vi "CmdControl _ch_1-12.vi"() -> (1 "Dataout":u8[](array[numeric]))   [LabVIEW 2017]
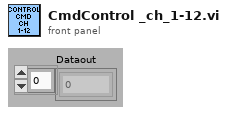
[diagram p1: front panel]
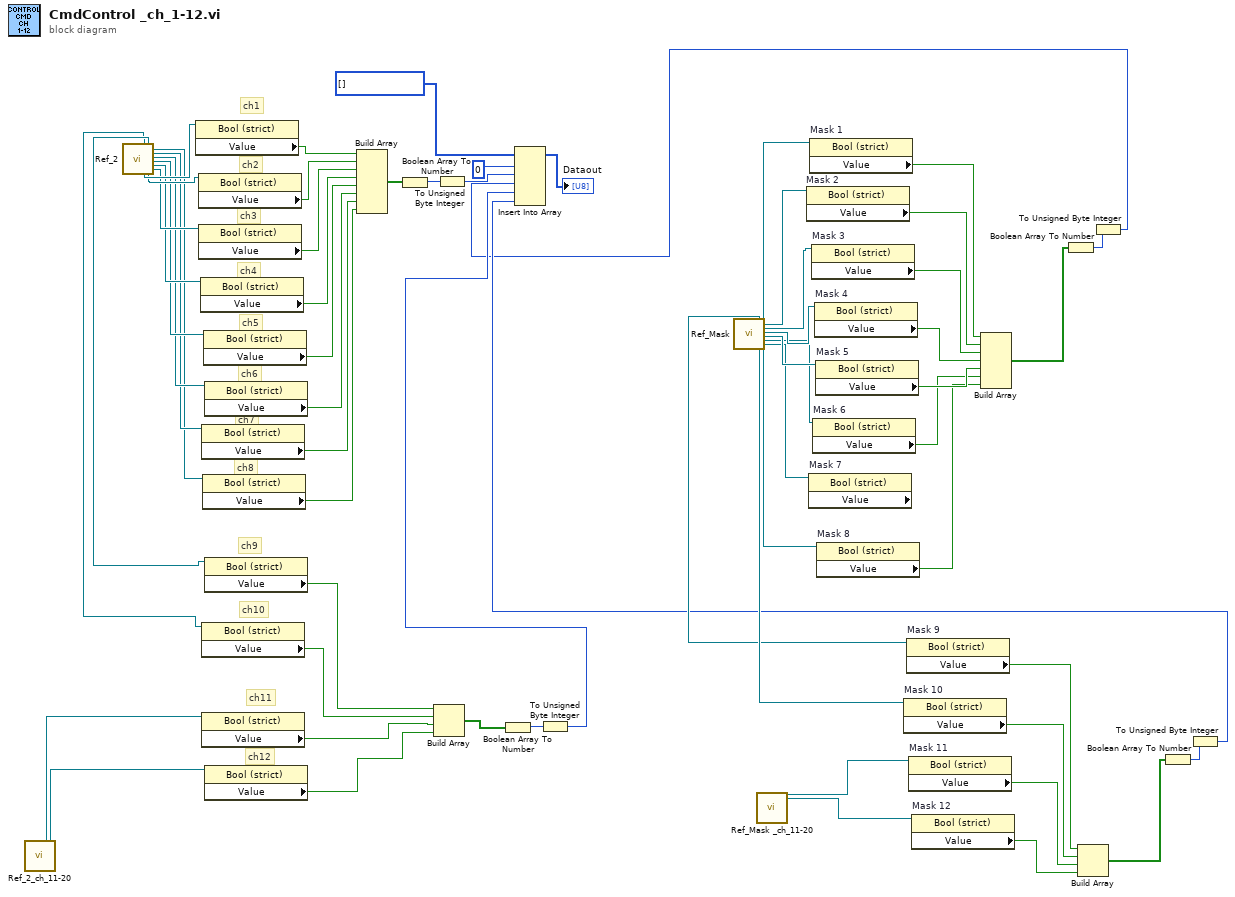
[diagram p0: block diagram]
diagram:
  # "ch12"
  # "ch11"
  # "ch10"
  # "ch9"
  # "ch8"
  # "ch7"
  # "ch6"
  # "ch5"
  # "ch4"
  # "ch3"
  # "ch2"
  # "ch1"
  n1 = call "Ref_2_ch_11-20.vi"() -> ("Control  Ch 11 out"=w37:refnum<vi>, "Control  Ch 12 out"=w38:refnum<vi>)  [unwired: 17 in, 9 out]
  n2 = call "Ref_2.vi"() -> ("Control  Ch 10 out"=w39:refnum<vi>, "Control  Ch 1 out"=w60:refnum<vi>, "Control  Ch 9 out"=w40:refnum<vi>, "Control  Ch 2 out"=w59:refnum<vi>, "Control  Ch 8 out"=w53:refnum<vi>, "Control  Ch 7 out"=w54:refnum<vi>, "Control  Ch 6 out"=w55:refnum<vi>, "Control  Ch 5 out"=w56:refnum<vi>, "Control  Ch 4 out"=w57:refnum<vi>, "Control  Ch 3 out"=w58:refnum<vi>)  [unwired: 17 in, 1 out]
  n3 = property class="Bool (strict)"(reference=w60) -> ("Value"=w52:bool)  [unwired: 1 in, 2 out]
  n4 = property class="Bool (strict)"(reference=w59) -> ("Value"=w51:bool)  [unwired: 1 in, 2 out]
  n5 = property class="Bool (strict)"(reference=w58) -> ("Value"=w50:bool)  [unwired: 1 in, 2 out]
  n6 = property class="Bool (strict)"(reference=w57) -> ("Value"=w49:bool)  [unwired: 1 in, 2 out]
  n7 = property class="Bool (strict)"(reference=w54) -> ("Value"=w46:bool)  [unwired: 1 in, 2 out]
  n8 = property class="Bool (strict)"(reference=w39) -> ("Value"=w35:bool)  [unwired: 1 in, 2 out]
  n9 = property class="Bool (strict)"(reference=w37) -> ("Value"=w34:bool)  [unwired: 1 in, 2 out]
  n10 = property class="Bool (strict)"(reference=w53) -> ("Value"=w45:bool)  [unwired: 1 in, 2 out]
  n11 = property class="Bool (strict)"(reference=w56) -> ("Value"=w48:bool)  [unwired: 1 in, 2 out]
  n12 = property class="Bool (strict)"(reference=w55) -> ("Value"=w47:bool)  [unwired: 1 in, 2 out]
  n13 = property class="Bool (strict)"(reference=w40) -> ("Value"=w36:bool)  [unwired: 1 in, 2 out]
  n14 = property class="Bool (strict)"(reference=w38) -> ("Value"=w33:bool)  [unwired: 1 in, 2 out]
  n15 = Build Array(w52, w51, w50, w49, w48, w47, w46, w45) -> (w44:bool[])
  n16 = Boolean Array To Number(Boolean array=w44) -> (number=w43:u32)
  n17 = Build Array(w36, w35, w34, w33) -> (w31:bool[])
  n18 = To Unsigned Byte Integer(number=w43) -> (unsigned 8bit integer=w42:u8)
  n19 = Boolean Array To Number(Boolean array=w31) -> (number=w32:u32)
  n20 = To Unsigned Byte Integer(number=w32) -> (unsigned 8bit integer=w30:u8)
  n21 = call "Ref_Mask.vi"() -> ("Mask Ch 9 out"=w5:refnum<vi>, "Mask Ch 10 out"=w6:refnum<vi>, "Mask Ch 1 out"=w21:refnum<vi>, "Mask Ch 2 out"=w20:refnum<vi>, "Mask Ch 3 out"=w19:refnum<vi>, "Mask Ch 4 out"=w18:refnum<vi>, "Mask Ch 5 out"=w17:refnum<vi>, "Mask Ch 6 out"=w16:refnum<vi>, "Mask Ch 7 out"=w15:refnum<vi>, "Mask Ch 8 out"=w14:refnum<vi>)  [unwired: 18 in]
  n22 = call "Ref_Mask _ch_11-20.vi"() -> ("Mask Ch 11 out"=w4:refnum<vi>, "Mask Ch 12 out"=w3:refnum<vi>)  [unwired: 18 in, 8 out]
  n23 = property on="Mask 2" class="Bool (strict)"(reference=w20) -> ("Value"=w26:bool)  [unwired: 1 in, 2 out]
  n24 = property on="Mask 7" class="Bool (strict)" props=["Value"](reference=w15) -> ()  [unwired: 1 in, 3 out]
  n25 = property on="Mask 1" class="Bool (strict)"(reference=w21) -> ("Value"=w27:bool)  [unwired: 1 in, 2 out]
  n26 = property on="Mask 3" class="Bool (strict)"(reference=w19) -> ("Value"=w25:bool)  [unwired: 1 in, 2 out]
  n27 = property on="Mask 6" class="Bool (strict)"(reference=w16) -> ("Value"=w22:bool)  [unwired: 1 in, 2 out]
  n28 = property on="Mask 4" class="Bool (strict)"(reference=w18) -> ("Value"=w24:bool)  [unwired: 1 in, 2 out]
  n29 = property on="Mask 5" class="Bool (strict)"(reference=w17) -> ("Value"=w23:bool)  [unwired: 1 in, 2 out]
  n30 = property on="Mask 8" class="Bool (strict)"(reference=w14) -> ("Value"=w13:bool)  [unwired: 1 in, 2 out]
  n31 = property on="Mask 10" class="Bool (strict)"(reference=w6) -> ("Value"=w9:bool)  [unwired: 1 in, 2 out]
  n32 = property on="Mask 9" class="Bool (strict)"(reference=w5) -> ("Value"=w10:bool)  [unwired: 1 in, 2 out]
  n33 = property on="Mask 11" class="Bool (strict)"(reference=w4) -> ("Value"=w8:bool)  [unwired: 1 in, 2 out]
  n34 = property on="Mask 12" class="Bool (strict)"(reference=w3) -> ("Value"=w7:bool)  [unwired: 1 in, 2 out]
  n35 = Build Array(w27, w26, w25, w24, w23, w22, w13) -> (w28:bool[])
  n36 = Boolean Array To Number(Boolean array=w28) -> (number=w29:u32)
  n37 = Build Array(w10, w9, w8, w7) -> (w11:bool[])
  n38 = To Unsigned Byte Integer(number=w29) -> (unsigned 8bit integer=w1:u8)
  n39 = Boolean Array To Number(Boolean array=w11) -> (number=w12:u32)
  n40 = To Unsigned Byte Integer(number=w12) -> (unsigned 8bit integer=w2:u8)
  n41 = Insert Into Array(array=u8[] [] ("Data 2"), index=0, new element #1=w42, new element #2=w1, new element #3=w30, new element #4=w2) -> (→"Dataout":u8[])
